vi "Synchronized Acquisition.vi"() -> ()   [LabVIEW 2021, in "GettingStarted_5774_Host.lvlib"]
uses:
  GettingStarted_5774_Host.lvlib
  <vilib>/userDefined/High Color/nirio_resource_hc.ctl
  <instrlib>/FlexRIO/API/Host/v1/NI FlexRIO/API/Reference Clock Source.ctl
  <vilib>/FPGAPlugInAG/Dynamic/niLvFpga_Reset_Dynamic.vi
  <vilib>/FPGAPlugInAG/Dynamic/niLvFpga_Run_Dynamic.vi
  <instrlib>/FlexRIO/API/Host/v1/NI FlexRIO/API/Configure Reference Clock.vi
  <instrlib>/FlexRIO/API/Host/v1/NI FlexRIO/API/Configure Immediate Start Trigger.vi
  <instrlib>/FlexRIO/API/Host/v1/NI FlexRIO/API/Configure Analog Start Trigger.vi
  <instrlib>/FlexRIO/API/Host/v1/NI FlexRIO/API/Configure Digital Edge Start Trigger.vi
  <instrlib>/FlexRIO/API/Host/v1/NI FlexRIO/API/Get Property Reference - Fpga Small.vi
  <instrlib>/FlexRIO/API/Host/v1/NI FlexRIO/API/Read Stream 1D WDT.vi
  <vilib>/FPGAPlugInAG/Dynamic/niLvFpga_Close_Dynamic.vi
  <vilib>/rvi/interface/nirviMethod/nirviMethod.xnode
  <vilib>/rvi/interface/nirviCloseFPGA/nirviCloseFPGA.xnode
  <instrlib>/FlexRIO/API/Host/v1/NI FlexRIO API v1.lvlib
  <resource>/objmgr/sessionReference.rc
  <resource>/objmgr/niflexrioapiStream.rc
panel:
  in  "reference clock source":T1 items=["Default", "Onboard", "PXI_Clk10", "External", "None", "Baseboard Reference"]
  in  "stop":bool
  out "error out":errorcluster
  out "Waveform Graph":waveform(dbl)[](graph)
  in  "acquire pretrigger \nsamples?":bool
  in  "min. TClk period":dbl=1e-06 format="%#_6p"
  in  "trigger master index":i32
  in  "Tab Control":enum32{"Immediate", "Digital", "Analog"}(tab)
  in  "trigger source":string(combo)="PXI_Trig0"
  in  "rising edge?":bool=TRUE
  in  "trigger channel":string="AI0"
  in  "level (V)":dbl
  in  "hysteresis (V)":dbl
  in  "device configuration":T3(array[cluster])=[{"FlexRIO digitizer"="RIO0", "channels"="AI0", "samples"=65536}, {"FlexRIO digitizer"="RIO1", "channels"="AI0", "samples"=65536}]
  # "Overview: Configure multiple FlexRIO targets for a synchronized acquisition using the FlexRIO Host API and NI-TClk API.\nRequirements: FlexRIO, NI-TClk\nInstructions: \n 1. Fill in the device configuration array with the resource name of the FlexRIO digitizers to synchronize, as well as the number of samples and which channels to acquire on.\n 2. Specify which device should be used as the trigger master using trigger master index\n 3. Configure the trigger settings for the master device\n 4. Optionally configure the reference clock to be used\n 5. Run the VI"
  # "Trigger Master Configuration"
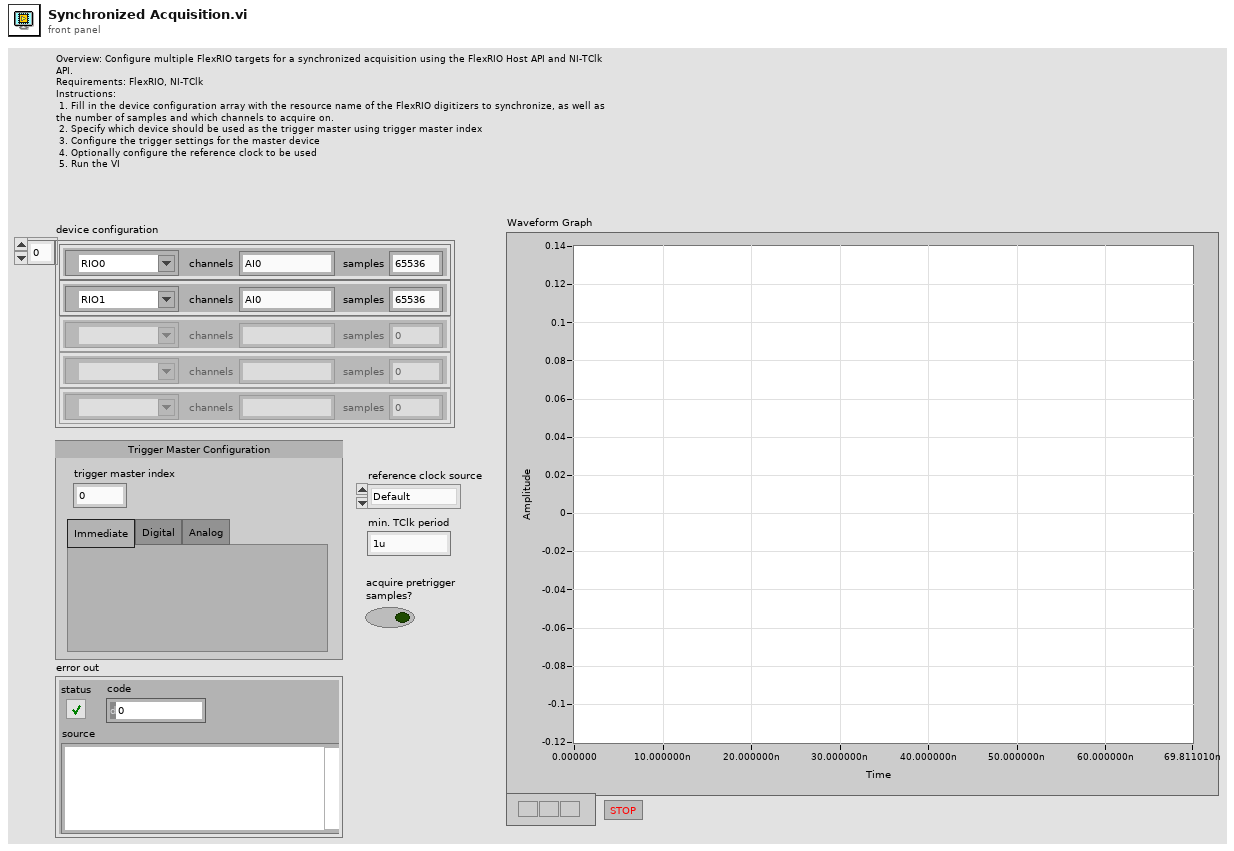
[diagram p1: front panel]
types:
  T1 = typedef "NI FlexRIO API v1.lvlib/Reference Clock Source.ctl" = i32
  T2 = typedef "nirio_resource_hc.ctl" = tag
  T3 = cluster{"FlexRIO digitizer":T2, "channels":string, "samples":u64}[]
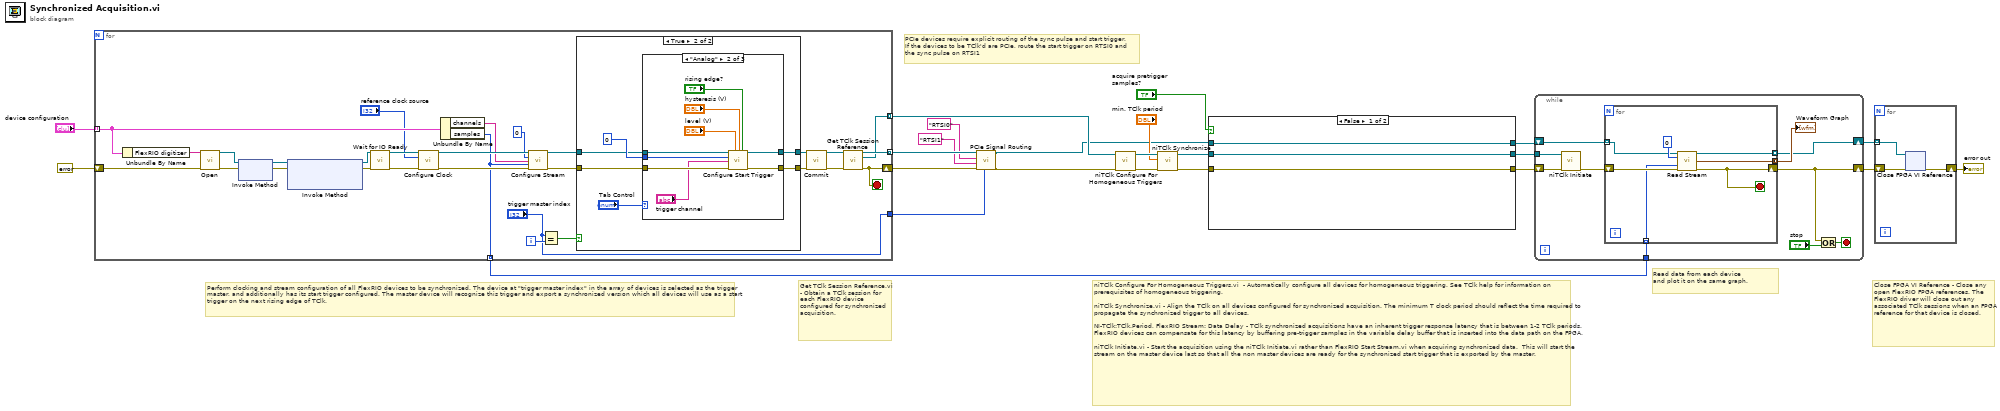
[diagram p0: block diagram]
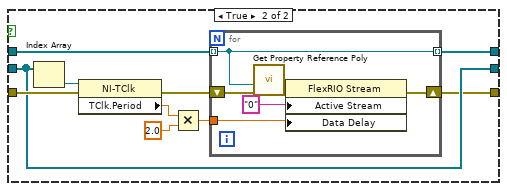
[diagram p2: hidden frame]
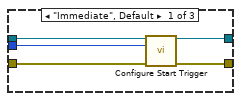
[diagram p4: hidden frame]
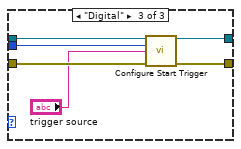
[diagram p5: hidden frame]
diagram:
  # "PCIe devices require explicit routing of the sync pulse and start trigger.\nIf the devices to be TClk'd are PCIe, route the start trigger on RTSI0 and\nthe sync pulse on RTSI1"
  # "Get TClk Session Reference.vi  - Obtain a TClk session for each FlexRIO device configured for synchronized acquisition."
  # "Perform clocking and stream configuration of all FlexRIO devices to be synchronized. The device at \"trigger master index\" in the array of devices is selected as the trigger master, and additionally has its start trigger configured. The master device will recognize this trigger and export a synchronized version which all devices will use as a start trigger on the next rising edge of TClk."
  # "niTClk Configure For Homogeneous Triggers.vi  - Automatically configure all devices for homogeneous triggering. See TClk help for information on prerequisites of homogeneous triggering. \n\nniTClk Synchronize.vi - Align the TClk on all devices configured for synchronized acquisition. The minimum T clock period should reflect the time required to propagate the synchronized trigger to all devices. \n\nNI-TClk:TClk.Period, FlexRIO Stream: Data Delay - TClk synchronized acquisitions have an inherent trigger response latency that is between 1-2 TClk periods. FlexRIO devices can compensate for this latency by buffering pre-trigger samples in the variable delay buffer that is inserted into the data path on the FPGA. \n\nniTClk Initiate.vi - Start the acquisition using the niTClk Initiate.vi rather than FlexRIO Start Stream.vi when acquiring synchronized data.  This will start the stream on the master device last so that all the non master devices are ready for the synchronized start trigger that is exported by the master."
  # "Read data from each device\nand plot it on the same graph."
  # "Close FPGA VI Reference - Close any open FlexRIO FPGA references. The FlexRIO driver will close out any associated TClk sessions when an FPGA reference for that device is closed."
  n1 = for {
    tunnel: "device configuration" -> [w45] mode=indexing
    tunnel: [w36] -> w6 mode=indexing
    tunnel: [w35] -> w11 mode=indexing
    shift-right: [w34] -> w7
    shift-left: errorcluster {"status"=FALSE, "code"=0, "source"=""} ("error out") -> [w33]
    tunnel: [w32] -> w14 mode=indexing
    tunnel: ["trigger master index"] -> w3
    i -> [w37]
    stop <- w34 stop-if-true
    n2 = Unbundle By Name(w45) -> ("FlexRIO digitizer"=w46:T2)
    n3 = call <instrlib>:"Open.vi"("RIO Device"=w46, "error in"=w33) -> ("fpga interface out"=w30:refnum<k20>, "error out"=w29:errorcluster)  [unwired: 12 in]
    n4 = xnode "Invoke Method"("FPGA VI Reference In"=w30, "error in"=w29) -> ("FPGA VI Reference Out"=w27:refnum<k20>, "error out"=w28:errorcluster)
    n5 = xnode "Invoke Method"("FPGA VI Reference In"=w27, "error in"=w28) -> ("FPGA VI Reference Out"=w25:refnum<k20>, "error out"=w26:errorcluster)  [unwired: 1 in]
    n6 = call <instrlib>:"Wait for IO Ready.vi"("fpga interface in"=w25, "error in"=w26) -> ("fpga interface out"=w52:refnum<k20>, "error out"=w51:errorcluster)  [unwired: 10 in, 2 out]
    n7 = call-poly <instrlib>:"Configure Clock.vi"("fpga interface in"=w52, "reference clock source"="reference clock source", "error in"=w51) -> ("fpga interface out"=w50:refnum<k20>, "error out"=w49:errorcluster)  [unwired: 11 in]
    n8 = Unbundle By Name(w45) -> ("channels"=w44:string, "samples"=w32:u64)
    n9 = call <instrlib>:"Configure Stream.vi"("fpga interface in"=w50, "stream instance"=u32 0, "channels enabled"=w44, "num samples"=w32, "error in"=w49) -> ("fpga interface out"=w47:refnum<k20>, "error out"=w48:errorcluster)  [unwired: 7 in, 2 out]
    n10 = Equal?(x="trigger master index", y=w37) -> (x = y?=w38:bool)
    n11 = case shown="True" w38 {
      tunnel: w48 -> [w53 w58]
      tunnel: w47 -> [w54 w57]
      tunnel: [w53 w56] -> w42
      tunnel: [w54 w55] -> w41
      frame False {
      }
      frame True {
        n12 = case shown="\"Analog\"" "Tab Control" {
          tunnel: w58 -> [w65 w74 w80]
          tunnel: [w64 w73 w79] -> w56
          tunnel: w57 -> [w63 w72 w78]
          tunnel: [w62 w71 w77] -> w55
          tunnel: u32 0 -> [w61 w70 w76]
          frame "Immediate", Default {
            n13 = call-poly <instrlib>:"Configure Start Trigger.vi"("fpga interface in"=w63, "trigger instance"=w61, "error in"=w65) -> ("fpga interface out"=w62:refnum<k20>, "error out"=w64:errorcluster)  [unwired: 10 in, 1 out]
          }
          frame "Analog" {
            n14 = call-poly <instrlib>:"Configure Start Trigger.vi"("fpga interface in"=w72, "level"="level (V)", "hysteresis"="hysteresis (V)", "rising edge?"="rising edge?", "trigger instance"=w70, "channel"="trigger channel", "error in"=w74) -> ("fpga interface out"=w71:refnum<k20>, "error out"=w73:errorcluster)  [unwired: 6 in, 1 out]
          }
          frame "Digital" {
            n15 = call-poly <instrlib>:"Configure Start Trigger.vi"("fpga interface in"=w78, "trigger instance"=w76, "trigger source"="trigger source", "error in"=w80) -> ("fpga interface out"=w77:refnum<k20>, "error out"=w79:errorcluster)  [unwired: 9 in, 1 out]
          }
        }
      }
    }
    n16 = call <instrlib>:"Commit.vi"("fpga interface in"=w41, "error in"=w42) -> ("fpga interface out"=w40:refnum<k20>, "error out"=w39:errorcluster)  [unwired: 12 in]
    n17 = call <instrlib>:"Get TClk Session Reference.vi"("fpga interface in"=w40, "error in"=w39) -> ("fpga interface out"=w36:refnum<k20>, "tclk session reference"=w35:refnum<k20>, "error out"=w34:errorcluster)  [unwired: 11 in]
  }
  n18 = call "PCIe Signal Routing.vi"("trigger master index"=w3, "error in"=w7, "sync pulse rtsi line"="RTSI1", "start trigger rtsi line"="RTSI0", "fpga interfaces in"=w6) -> ("error out"=w1:errorcluster, "fpga interfaces out"=w2:refnum<k20>[])  [unwired: 5 in]
  n19 = call <instrlib>:"niTClk Configure For Homogeneous Triggers.vi"("error in (no error)"=w1, "sessions"=w11) -> ("error out"=w22:errorcluster, "sessions out"=w21:refnum<k20>[])  [unwired: 8 in]
  n20 = call <instrlib>:"niTClk Synchronize.vi"("error in (no error)"=w22, "minimum T clock period"="min. TClk period", "sessions"=w21) -> ("error out"=w20:errorcluster, "sessions out"=w19:refnum<k20>[])  [unwired: 7 in]
  n21 = case shown="False" "acquire pretrigger \nsamples?" {
    tunnel: w2 -> [w83 w92]
    tunnel: [w83 w91] -> w9
    tunnel: w20 -> [w81 w90]
    tunnel: w19 -> [w82 w86]
    tunnel: [w82 w86] -> w10
    tunnel: [w81 w85] -> w18
    frame False {
    }
    frame True {
      n22 = Index Array(array=w86) -> (element=w93:refnum<k20>)  [unwired: 1 in]
      n23 = property class="NI-TClk"(reference=w93, error in=w90) -> (error out=w84:errorcluster, "TClk.Period"=w88:dbl)  [unwired: 1 out]
      n24 = Multiply(x=w88, y=2.0) -> (x*y=w87:dbl)
      n25 = for {
        tunnel: w92 -> [w94] mode=indexing
        tunnel: [w94] -> w91 mode=indexing
        tunnel: w87 -> [w98]
        shift-right: [w97] -> w85
        shift-left: w84 -> [w96]
        n26 = call-poly <instrlib>:"Get Property Reference Poly.vi"("error in (no error)"=w96, "fpga interface in"=w94) -> ("error out"=w95:errorcluster, "property reference"=w100:refnum<k20>)  [unwired: 4 in, 1 out]
        n27 = property class="FlexRIO Stream"(reference=w100, error in=w95, "Active Stream"="0", "Data Delay"=w98) -> (error out=w97:errorcluster)  [unwired: 1 out]
      }
    }
  }
  n28 = while {
    tunnel: w10 -> [w110]
    tunnel: w14 -> [w106]
    shift-right: [w101] -> w13
    shift-left: w18 -> [w109]
    shift-right: [w104] -> w8
    shift-left: w9 -> [w108]
    stop <- w103 stop-if-true
    n29 = call <instrlib>:"niTClk Initiate.vi"("error in (no error)"=w109, "sessions"=w110) -> ("error out"=w107:errorcluster)  [unwired: 8 in, 1 out]
    n30 = for {
      tunnel: w108 -> [w115] mode=indexing
      shift-right: [w111] -> w101
      shift-left: w107 -> [w116]
      tunnel: w106 -> [w114] mode=indexing
      tunnel: [w113] -> w104 mode=indexing
      tunnel: [w112] -> w105 mode=concatenating
      stop <- w111 stop-if-true
      n31 = call-poly <instrlib>:"Read Stream.vi"("fpga interface in"=w115, "stream instance"=u32 0 ("stream number"), "samples"=w114, "error in"=w116) -> ("fpga interface out"=w113:refnum<k20>, "read data"=w112:waveform(dbl)[], "error out"=w111:errorcluster)  [unwired: 7 in, 2 out]
    }
    "Waveform Graph" <- w105
    n32 = Or(x=w101, y="stop") -> (x .or. y?=w103:bool)
  }
  n33 = for {
    tunnel: w8 -> [w119] mode=indexing
    shift-right: [w118] -> w12
    shift-left: w13 -> [w120]
    n34 = xnode "Close FPGA VI Reference"("FPGA VI Reference In"=w119, "error in"=w120) -> ("error out"=w118:errorcluster)
  }
  "error out" <- w12
